vi "TEST LS-335.vi"() -> ()   [LabVIEW 2017]
uses:
  LS-335 SET PID.ctl
  LS-335_Hardware_Module Control.ctl
panel:
  in  "PID Settings":T1={"Heater Output (1:1)"=1, "Gain (P) (50.0)"=50.0, "Reset (I) (20.0)"=20.0, "Rate (D) (0.0 %)"=0.0, "Range (0:Off)"=0, "Manual Output (0.00 %)"=0.0} {"Heater Output (1:1)" items=["1"=1, "2"=2]; "Range (0:Off)" items=["Off", "Low (On)", "Medium", "High"]; "Manual Output (0.00 %)" format="%.2f"; "Rate (D) (0.0 %)" format="%.1f"; "Reset (I) (20.0)" format="%.1f"; "Gain (P) (50.0)" format="%.1f"}
  in  "Ramp Rate (0.0)":dbl format="%.1f"
  in  "Setpoint (0.0000)":dbl format="%.4f"
  in  "PID-POWER":bool
  in  "SETPOINT":bool
  out "Waveform Chart":dbl(graph)
  out "error out":errorcluster
  in  "stop":bool
  # "LAKE SHORE MODEL 335 TEST PANEL"
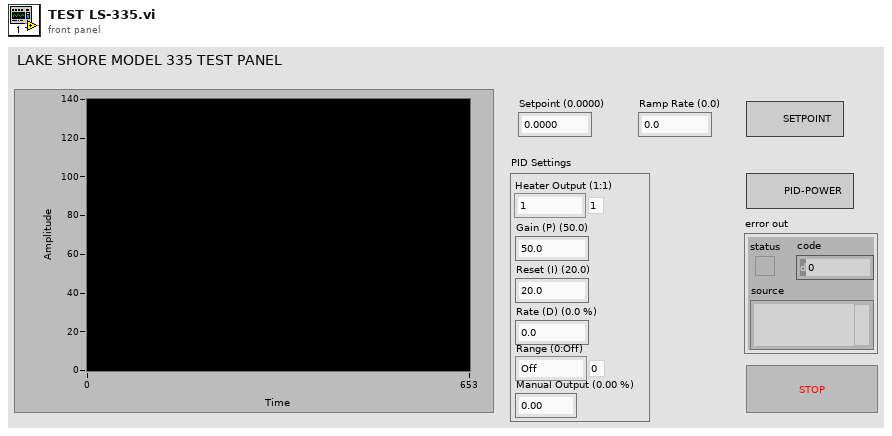
[diagram p1: front panel]
types:
  T1 = typedef "LS-335 SET PID.ctl" = cluster{"Heater Output (1:1)":u16, "Gain (P) (50.0)":dbl, "Reset (I) (20.0)":dbl, "Rate (D) (0.0 %)":dbl, "Range (0:Off)":u16, "Manual Output (0.00 %)":dbl}
  T2 = typedef "LS-335_Hardware_Module Control.ctl" = enum16{"INITIALIZE", "READ TEMPERATURE", "READ CONTROL DATA", "WRITE SETPOINT AND RATE", "WRITE PID AND POWER RANGE", "WRITE CONTROL PARAMETERS", "SHUTDOWN"}
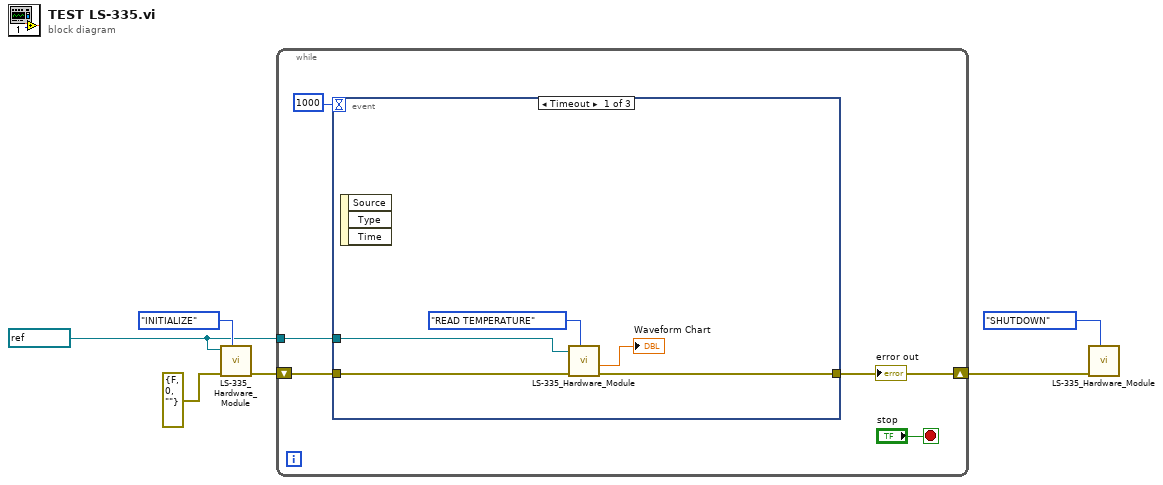
[diagram p0: block diagram]
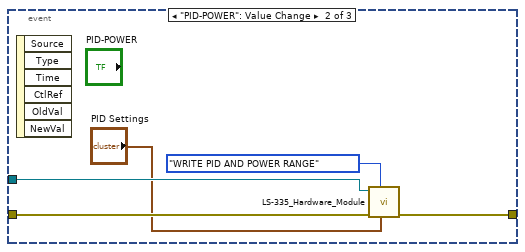
[diagram p2: hidden frame]
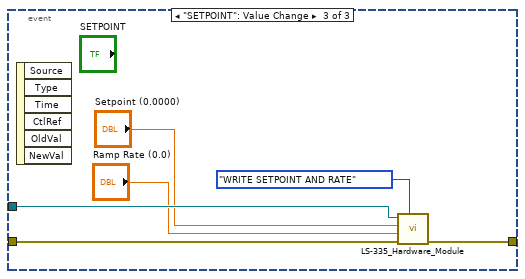
[diagram p3: hidden frame]
diagram:
  w1 = refnum<visa-resource-name> "COM3" ("VISA resource name")
  n1 = call "LS-335_Hardware_Module.vi"("Command"=LS-335_Hardware_Module_Control."INITIALIZE", "error in (no error)"=errorcluster {"status"=FALSE, "code"=0, "source"=""}, "VISA resource name"=w1) -> ("error out"=w5:errorcluster)  [unwired: 7 in, 1 out]
  n2 = while {
    shift-right: [w9] -> w4
    shift-left: w5 -> [w10]
    tunnel: w1 -> [w7]
    stop <- "stop" stop-if-true
    n3 = event shown="[0] Timeout" {
      selector: _ -> [_ _ _]
      dyn-events: _ -> [_ _ _]
      timeout: 1000 -> [_ _ _]
      tunnel: w10 -> [w15 w19 w22]
      tunnel: [w13 w20 w26] -> w9
      tunnel: w7 -> [w14 w18 w25]
      event Timeout {
        n4 = event-data() -> ()  [unwired: 1 in, 3 out]
        n5 = call "LS-335_Hardware_Module.vi"("Command"=LS-335_Hardware_Module_Control."READ TEMPERATURE", "error in (no error)"=w15, "VISA resource name"=w14) -> ("error out"=w13:errorcluster, "Sensor Data"=→"Waveform Chart":dbl)  [unwired: 7 in]
      }
      event "PID-POWER": Value Change {
        n6 = event-data() -> ()  [unwired: 1 in, 6 out]
        n7 = call "LS-335_Hardware_Module.vi"("PID Settings"="PID Settings", "Command"=LS-335_Hardware_Module_Control."WRITE PID AND POWER RANGE", "error in (no error)"=w19, "VISA resource name"=w18) -> ("error out"=w20:errorcluster)  [unwired: 6 in, 1 out]
      }
      event "SETPOINT": Value Change {
        n8 = event-data() -> ()  [unwired: 1 in, 6 out]
        n9 = call "LS-335_Hardware_Module.vi"("Command"=LS-335_Hardware_Module_Control."WRITE SETPOINT AND RATE", "error in (no error)"=w22, "Ramp Rate (0.0)"="Ramp Rate (0.0)", "Setpoint (0.0000)"="Setpoint (0.0000)", "VISA resource name"=w25) -> ("error out"=w26:errorcluster)  [unwired: 5 in, 1 out]
      }
    }
    "error out" <- w9
  }
  n10 = call "LS-335_Hardware_Module.vi"("Command"=LS-335_Hardware_Module_Control."SHUTDOWN", "error in (no error)"=w4) -> ()  [unwired: 8 in, 2 out]
